vi "MainProgram.vi"() -> ()   [LabVIEW 2015]
uses:
  Semaphores ring.ctl
  Separated VIs/ColorSensors Enum.ctl
  <vilib>/NXT/Subs/ColorSensorColors.ctl
  <vilib>/NXT/Block Support/NXT_InputPort.ctl
  <vilib>/NXT/Block Support/NXT_ButtonSelector.ctl
  Separated VIs/Behavior number ring.ctl
  <vilib>/NXT/Subs/MotorOutput.ctl
  <vilib>/NXT/Block Support/NXT_OutputPort.ctl
  <vilib>/NXT/Dual Mode Library/Advanced/NXTFlag_Assign.vi
  <vilib>/NXT/Dual Mode Library/Advanced/NXTFlag_Get.vi
  <vilib>/NXT/Dual Mode Library/Sensors/Color_Detector.vi
  <vilib>/NXT/Dual Mode Library/Sensors/Sonar_cm.vi
  <vilib>/NXT/Dual Mode Library/Display/drawNumber.vi
  <vilib>/NXT/Dual Mode Library/Sound/Tone.vi
  <vilib>/NXT/NXTIO Xnodes/NXTIONodeSubVIs/NXTMoveMotors.vi
  <vilib>/NXT/NXTIO Xnodes/NXTIONodeSubVIs/NXTStopMotors.vi
  <vilib>/NXT/Dual Mode Library/Waits/Wait_Num.vi
  <vilib>/NXT/Dual Mode Library/Sensors/Touch_Pressed.vi
  <vilib>/NXT/NXTIO Xnodes/NXTIONodeSubVIs/NXTMotorRunDistance.vi
  <vilib>/NXT/NXTIO Xnodes/NXTIONodeSubVIs/NXTMotorSteeringOn.vi
  <vilib>/NXT/Dual Mode Library/Motors/MotorBrake.vi
  <vilib>/NXT/Dual Mode Library/Advanced/NXTFlag_Clear.vi
  <vilib>/NXT/Dual Mode Library/Sensors/readNXTButton.vi
  <vilib>/NXT/NXTIO Xnodes/AddressXNode/NXTIOAddress.xnode
  <vilib>/NXT/NXTIO Xnodes/NXTIOXNode/NXTIO.xnode
  <vilib>/NXT/Subs/LVHSConnector.ctl
  <vilib>/NXT/LegoClasses/BrickReference/BrickReference.lvclass
panel:
  out "Wander Angle":i32
  out "Wander Time":i32
  out "Wander Direction":u16(ring) items=["right", "left"]
  out "Wander Speed":i32
  in  "Behavior Wire In":T1
  in  "Max Behavior Number":i32=8
  in  "Behavior Wires In":T2(array[cluster])
  out "Behavior Wire Output":T1
  out "Behavior Required Found Flag":bool
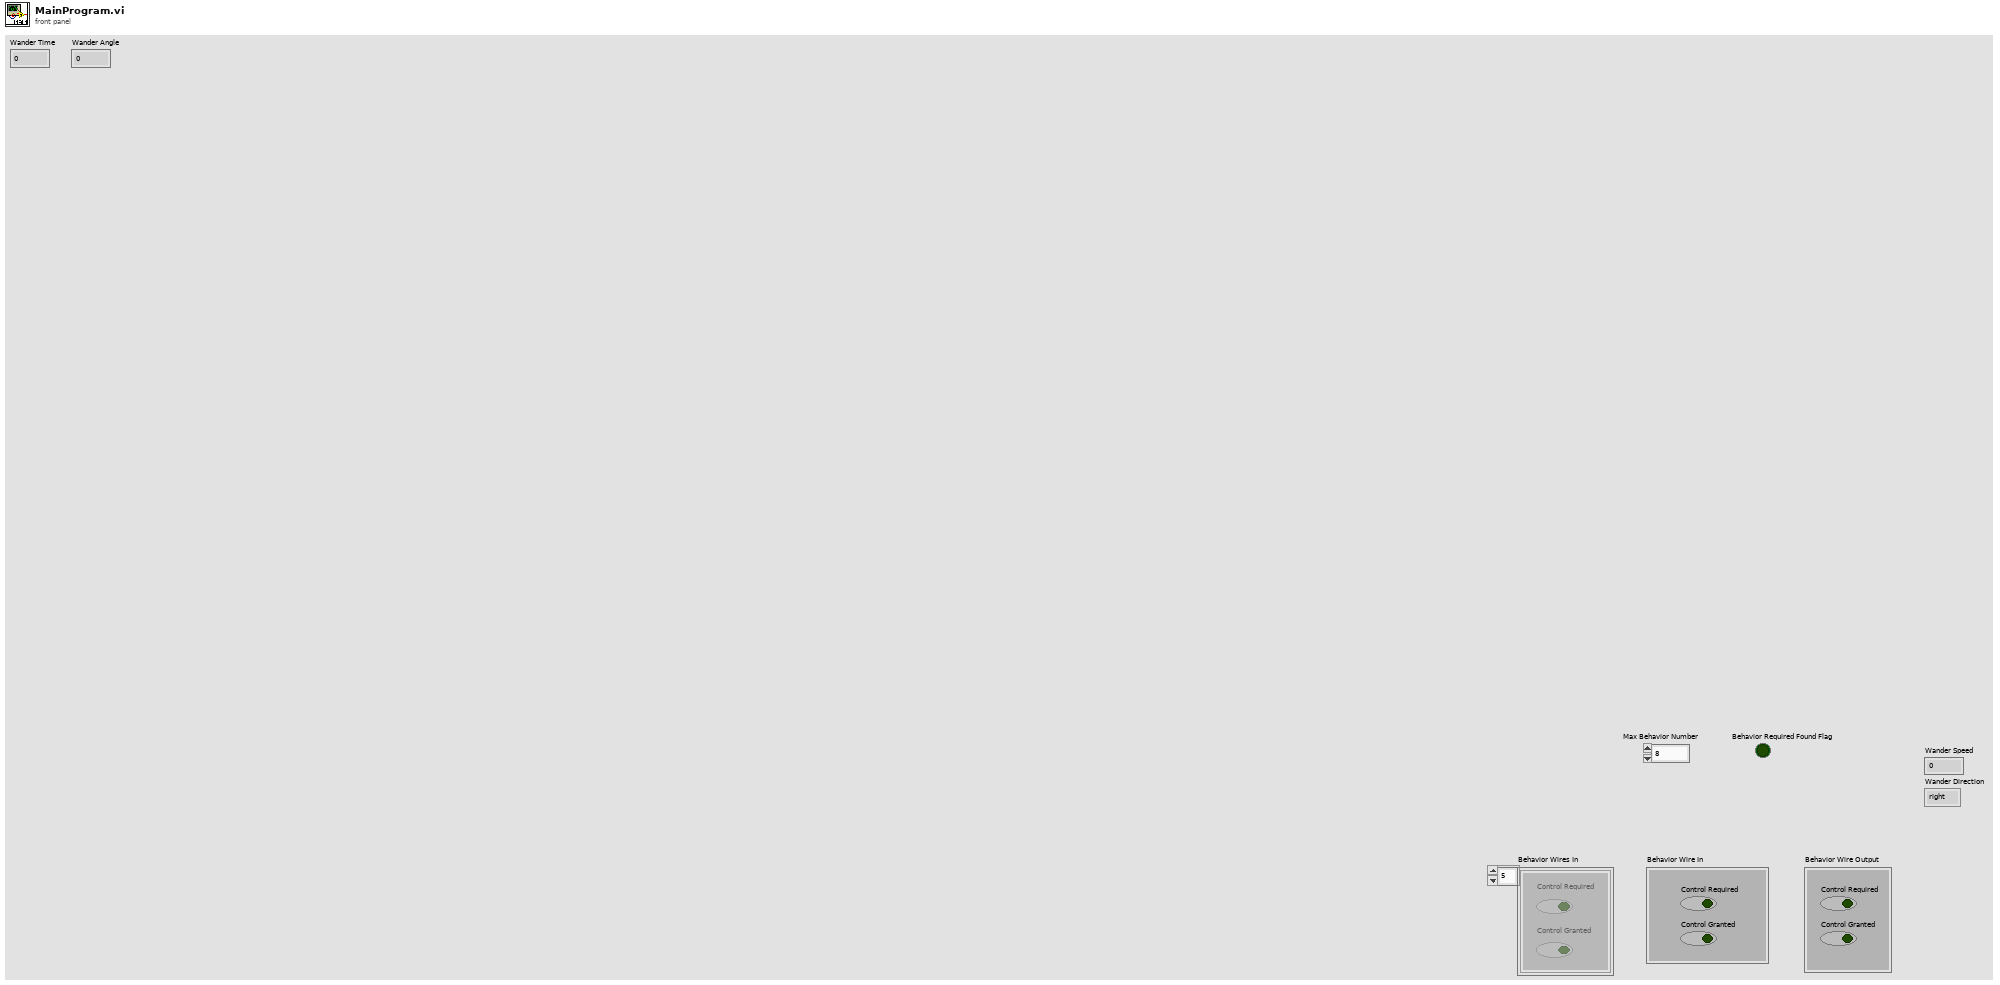
[diagram p1: front panel]
types:
  T1 = cluster{"Control Required":bool, "Control Granted":bool}
  T2 = cluster{"Control Required":bool, "Control Granted":bool}[]
  T3 = typedef "ColorSensors Enum.ctl" = enum16{"Not Recognised", "Black", "Blue", "Green", "Yellow", "Red", "White"}
  T4 = typedef "NXT_OutputPort.ctl" = u8
  T5 = typedef "ColorSensorColors.ctl" = enum16{"No Color", "Black", "Blue", "Green", "Yellow", "Red", "White", "Brown"}
  T6 = typedef "Semaphores ring.ctl" = u16
  T7 = typedef "LVHSConnector.ctl" = refnum<class "BrickReference.lvclass">
  T8 = typedef "NXT_InputPort.ctl" = u32
  T9 = typedef "Behavior number ring.ctl" = u16
  T10 = typedef "MotorOutput.ctl" = u8
  T11 = typedef "NXT_ButtonSelector.ctl" = u16
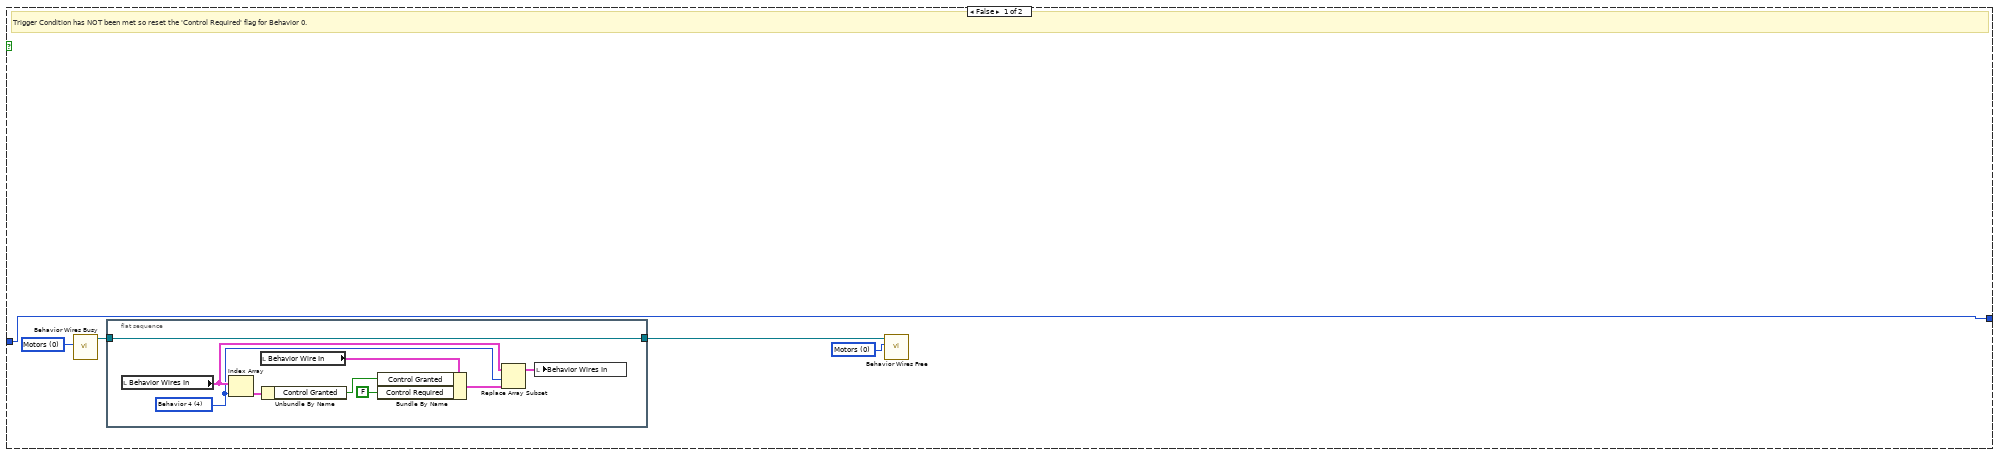
[diagram p3: hidden frame]
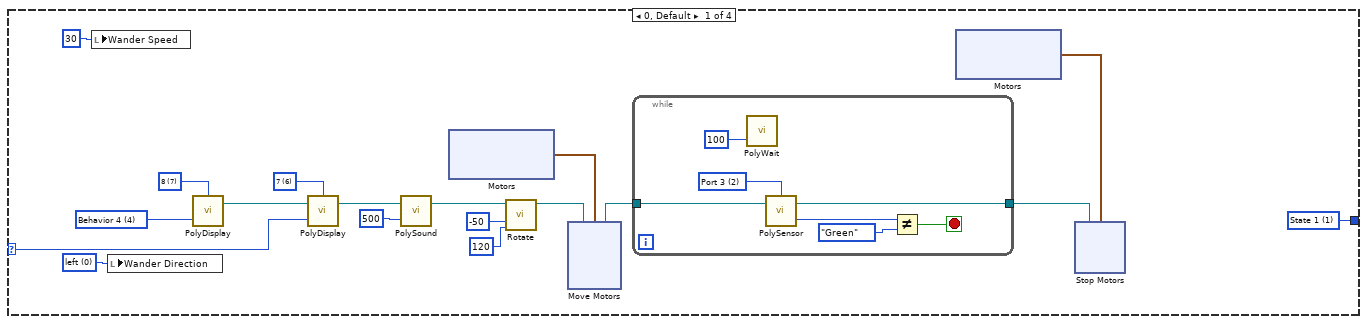
[diagram p5: hidden frame]
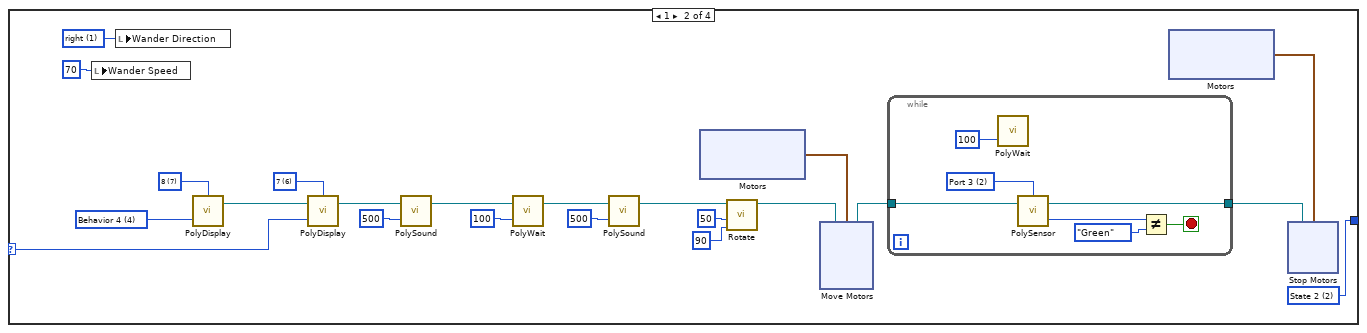
[diagram p6: hidden frame]
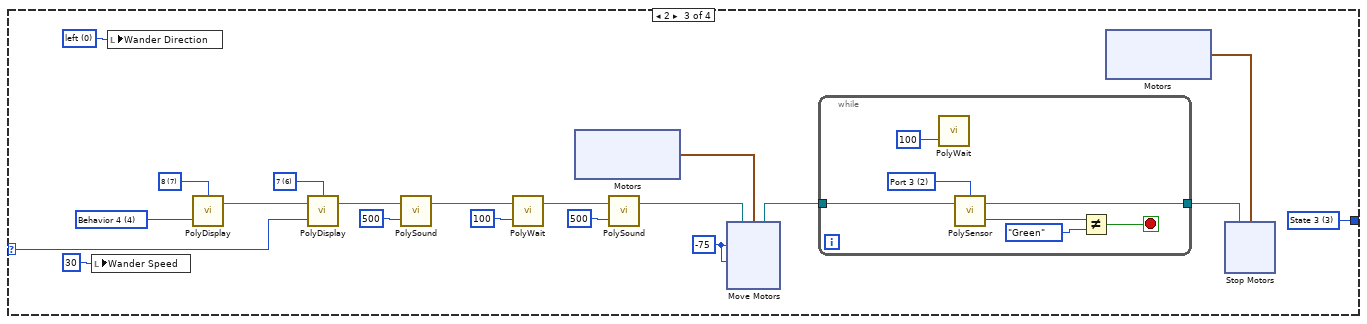
[diagram p7: hidden frame]
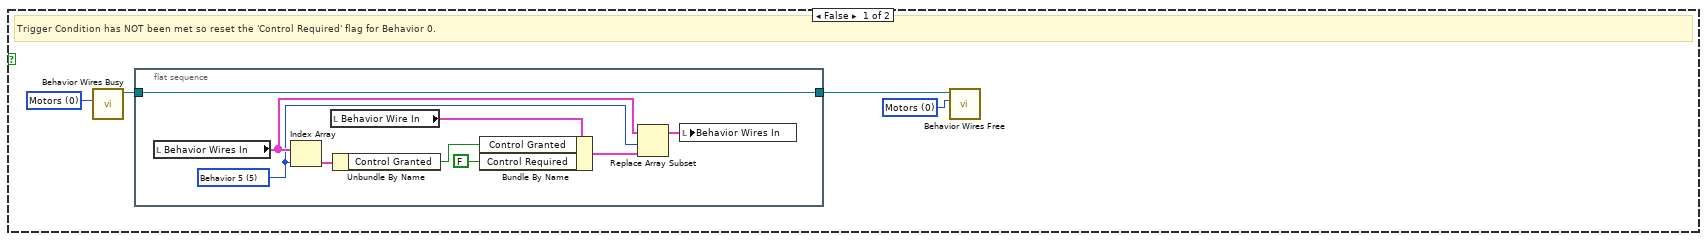
[diagram p8: hidden frame]
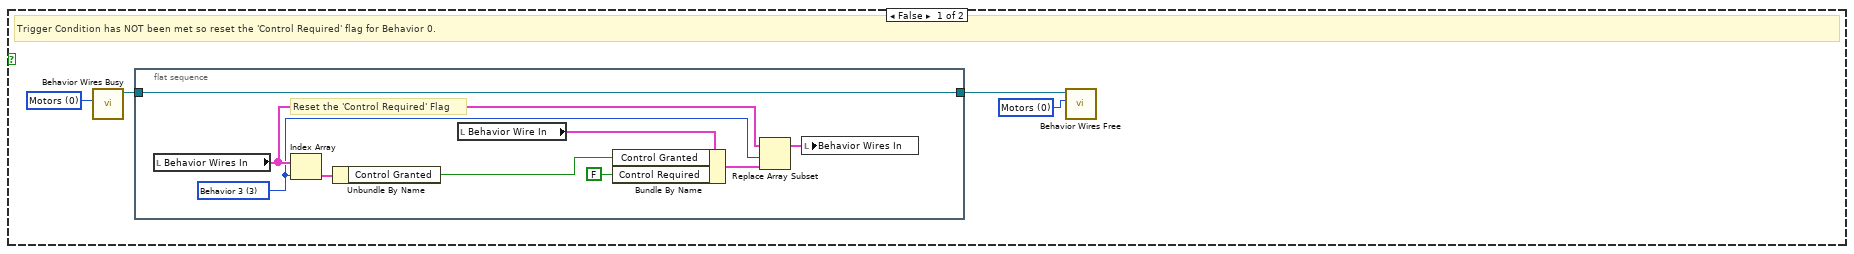
[diagram p10: hidden frame]
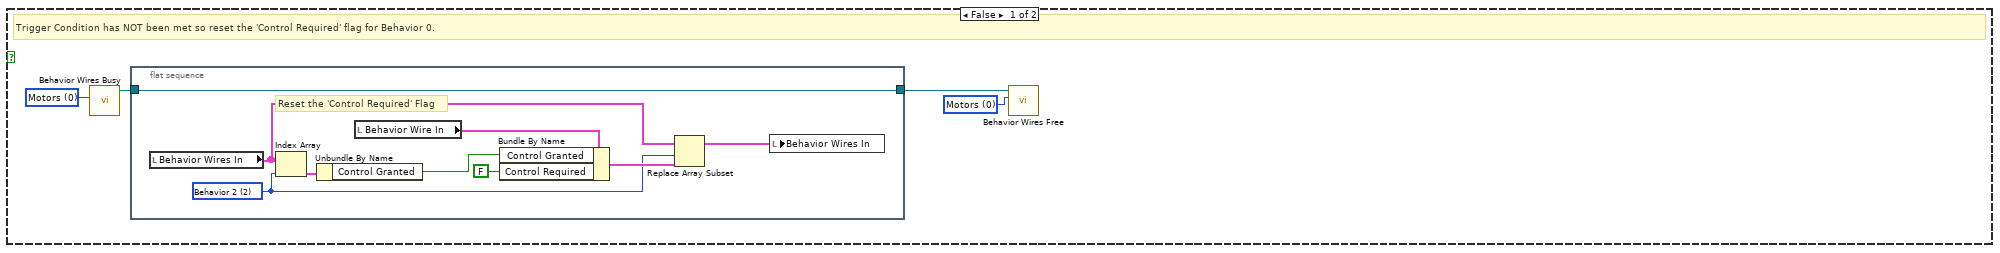
[diagram p12: hidden frame]
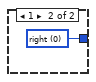
[diagram p14: hidden frame]
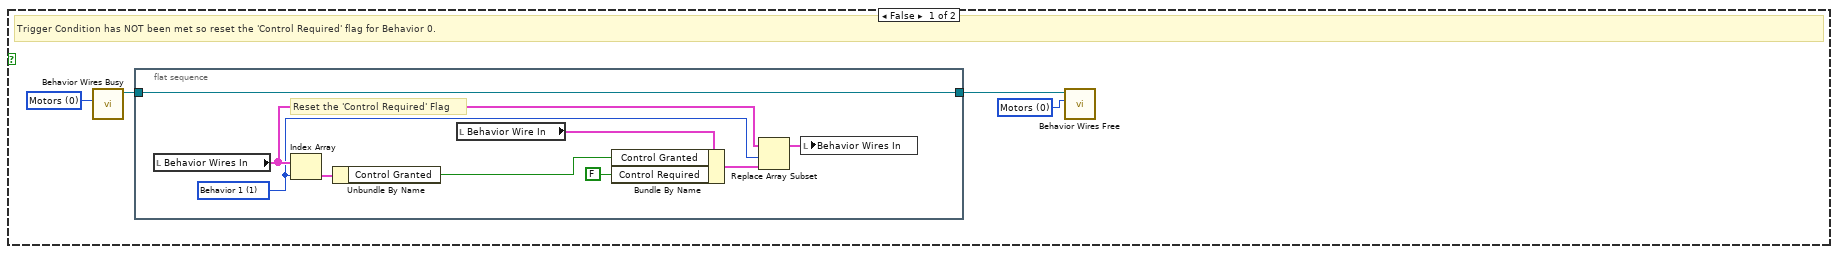
[diagram p15: hidden frame]
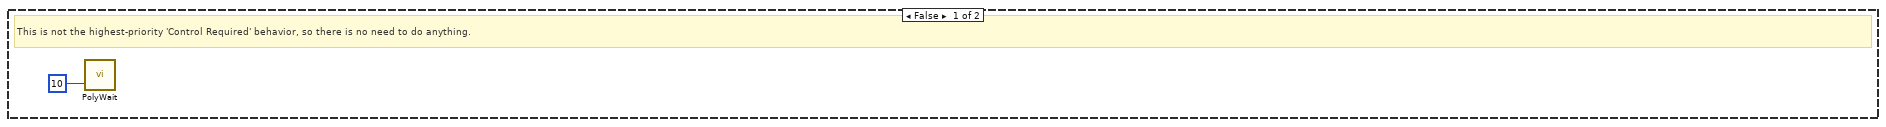
[diagram p17: hidden frame]
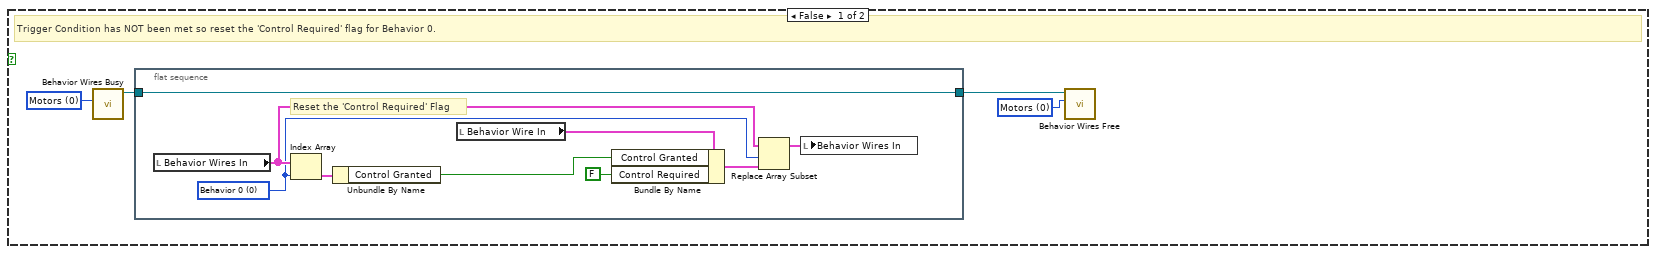
[diagram p20: hidden frame]
diagram:
  n1 = flat-sequence {
    tunnel: [w7] -> w2
    tunnel: w2 -> [w17]
    tunnel: [w18] -> w1
    tunnel: w1 -> [w666]
    frame #0 {
      w5 = u16 1 items=["right", "left"] ("Ring")
      # "Step 1 : Housekeeping\n\nInitalise the Wires array (to False) and \nset the semaphore to begin operation"
      n2 = flat-sequence {
        tunnel: [w13] -> w7
        frame #0 {
          n3 = Initialize Array("Behavior Wire In", "Max Behavior Number") -> (w8:T2)
          n4 = local write "Behavior Wires In"(w8) -> ()
        }
        frame #1 {
          w11 = T6 0 items=["Motors", "Exit", "Sonar"] ("Semaphores")
          w12 = T6 1 items=["Motors", "Exit", "Sonar"] ("Semaphores")
          n5 = call "Behavior Wires Free.vi"("Semaphore Number"=w11) -> ("Sequence Out"=w14:T7)  [unwired: 9 in]
          n6 = call-poly <vilib>:"NXTFlag_Assign_Poly.vi"("Flag State"=FALSE, "NXT/EV3"=w14, "NXT/EV3 Flag Number"=w12) -> ("NXT/EV3"=w13:T7)  [unwired: 1 in]
        }
      }
      "Wander Speed" <- 30
      "Wander Direction" <- w5
      "Wander Time" <- 8
      "Wander Angle" <- 60
    }
    frame #1 {
      w16 = u16 0 items=["State 0", "State 1", "State 2", "State 3"] ("Ring")
      # "Step 2: Execute the behaviors until shutdown is initiated\n                                       \nThe behaviors are placed in separate  parallel loops. \nAccess to the wire cluster array is controlled using a semaphore flag (Contained in 'Behavior Wires Busy' and 'Behavior Wires Free' VIs.. ).\nNote, When 'Behavior Wires Busy' is called, access by the arbiter is suspended,  so it is important that  'Behavior Wires Free' is always called as soon as possible afterwards.\n\nNote: You cannot make a subVI of the Wire operations. The simplified memory manager can't deal with the re-direction.\n\nTo use this example: Behavior 1 - drives in a straight line, Behavior 2 - Sonar at 25 cms rotates and drives off and Behavior 3 - bump sensor causes robot to reverse and pivot"
      n7 = while {
        stop <- w541 stop-if-true
        w540 = T6 1 items=["Motors", "Exit", "Sonar"] ("Semaphores")
        # "Arbiter - Scans all the behaviors to determine which behvior has the highest priority (higher value higher priority). \nCheck from largest index down for 'Control required' Flag set. If first encounter of set flag, set 'Control Granted' flag for behavior.\nReset all lower 'Control Granted' behavior Flags. If no 'Control Required flag' set, reset the resource values"
        n8 = flat-sequence {
          frame #0 {
            # "Reset the 'Behavior Required Found' flag\n before searching..."
            n9 = local write "Behavior Required Found Flag"(FALSE) -> ()
          }
          frame #1 {
            # "... searching for the highest-priority behavior looking for control (i.e. currently with 'Control Required' flag set)."
            n10 = local read "Max Behavior Number"() -> (w543:i32)
            n11 = for {
              N: w543 -> [_]
              i -> [w554]
              n12 = local read "Max Behavior Number"() -> (w545:i32)
              n13 = local read "Behavior Required Found Flag"() -> (w551:bool)
              n14 = local read "Behavior Wires In"() -> (w553:T2)
              n15 = Subtract(x=w545, y=1) -> (x-y=w546:i32)
              n16 = Subtract(x=w546, y=w554) -> (x-y=w549:i32)
              n17 = Index Array(array=w553, index=w549) -> (element=w552:T1)
              n18 = Unbundle By Name(w552) -> ("Control Required"=w548:bool)
              n19 = Not(x=w551) -> (.not. x?=w547:bool)
              n20 = And(x=w547, y=w548) -> (x .and. y?=w550:bool)
              n21 = case shown="True" w550 {
                tunnel: w549 -> [_ w557]
                frame False {
                  # "This is not the highest-priority 'Control Required' behavior, so there is no need to do anything."
                  n22 = call-poly <vilib>:"PolyWait.vi"("Time (100 msec)"=u32 10) -> ()  [unwired: 3 in, 1 out]
                }
                frame True {
                  # "This IS the highest priority 'Control Required' flag"
                  n23 = flat-sequence {
                    tunnel: w557 -> [w563]
                    tunnel: [w563] -> w556
                    tunnel: w556 -> [w569]
                    frame #0 {
                      w558 = T6 0 items=["Motors", "Exit", "Sonar"] ("Semaphores")
                      w559 = T6 0 items=["Motors", "Exit", "Sonar"] ("Semaphores")
                      # "Set the highest 'Control Granted' and 'Behavior Required Found Flag's to True"
                      n24 = flat-sequence {
                        tunnel: w563 -> [w565]
                        tunnel: w561 -> [w564]
                        tunnel: [w564] -> w560
                        frame #0 {
                          n25 = local read "Behavior Wires In"() -> (w567:T2)
                          n26 = Replace Array Subset(array=w567, new element=T1 {"Control Required"=TRUE, "Control Granted"=TRUE} ("Behavior Wire In"), index=w565) -> (w568:T2)
                          n27 = local write "Behavior Wires In"(w568) -> ()
                        }
                      }
                      n28 = local write "Behavior Required Found Flag"(TRUE ("Behavior Required Found Flag")) -> ()
                      n29 = call "Behavior Wires Busy.vi"("Semaphore Number"=w559) -> ("Sequence Out"=w561:T7)  [unwired: 9 in]
                      n30 = call "Behavior Wires Free.vi"("Sequence In"=w560, "Semaphore Number"=w558) -> ()  [unwired: 8 in, 1 out]
                    }
                    frame #1 {
                      # "...And reset all lower 'Control Granted' Flags"
                      n31 = for {
                        N: w569 -> [_]
                        tunnel: w569 -> [w572]
                        i -> [w570]
                        n32 = Not Equal?(x=w572, y=w570) -> (x != y?=w571:bool)
                        n33 = case shown="True" w571 {
                          tunnel: w570 -> [_ w575]
                          frame False {
                            # "This is the highest priority index so DO NOT reset the 'Control Granted' flag."
                          }
                          frame True {
                            w573 = T6 0 items=["Motors", "Exit", "Sonar"] ("Semaphores")
                            w574 = T6 0 items=["Motors", "Exit", "Sonar"] ("Semaphores")
                            # "This is NOT the highest priority index so DO reset the 'Control Granted' flag."
                            n34 = call "Behavior Wires Busy.vi"("Semaphore Number"=w574) -> ("Sequence Out"=w576:T7)  [unwired: 9 in]
                            n35 = flat-sequence {
                              tunnel: w575 -> [w579]
                              tunnel: [w578] -> w577
                              tunnel: w576 -> [w578]
                              frame #0 {
                                # "Reset 'Control Granted' flag for remaining behaviors"
                                n36 = local read "Behavior Wires In"() -> (w584:T2)
                                n37 = Index Array(array=w584, index=w579) -> (element=w582:T1)
                                n38 = Unbundle By Name(w582) -> ("Control Required"=w581:bool)
                                n39 = local read "Behavior Wire In"() -> (w583:T1)
                                n40 = Bundle By Name(cluster=w583, "Control Required"=w581, "Control Granted"=FALSE) -> (w585:T1)
                                n41 = Replace Array Subset(array=w584, new element=w585, index=w579) -> (w586:T2)
                                n42 = local write "Behavior Wires In"(w586) -> ()
                              }
                            }
                            n43 = call "Behavior Wires Free.vi"("Sequence In"=w577, "Semaphore Number"=w573) -> ()  [unwired: 8 in, 1 out]
                          }
                        }
                      }
                    }
                  }
                }
              }
            }
          }
        }
        n44 = call-poly <vilib>:"NXTFlag_Get_Poly.vi"("NXT/EV3 Flag Number"=w540) -> ("status"=w541:bool)  [unwired: 2 in, 1 out]
      }
      n45 = while {
        stop <- w482 stop-if-true
        w473 = T8 3 items=["Port 1", "Port 2", "Port 3", "Port 4"] ("Port (Port 4)")
        w474 = T8 2 items=["Port 1", "Port 2", "Port 3", "Port 4"] ("Port (Port 3)")
        w481 = T6 1 items=["Motors", "Exit", "Sonar"] ("Semaphores")
        # "No color -> Change to some color"
        # "Behavior 1"
        n46 = call-poly <vilib>:"PolySensor.vi"("Port (Port 3)"=w474) -> ("Detected Color"=w480:T5)  [unwired: 2 in, 1 out]
        n47 = call-poly <vilib>:"PolySensor.vi"("Port (Port 4)"=w473) -> ("Distance (cm)"=w477:i16)  [unwired: 2 in, 1 out]
        n48 = Equal?(x=w480, y=ColorSensorColors."White") -> (x = y?=w478:bool)
        n49 = Less?(x=w477, y=i16 10) -> (x < y?=w475:bool)
        n50 = And(x=w475, y=w478) -> (x .and. y?=w472:bool)
        n51 = case shown="True" w472 {
          frame False {
            w483 = T6 0 items=["Motors", "Exit", "Sonar"] ("Semaphores")
            w484 = T6 0 items=["Motors", "Exit", "Sonar"] ("Semaphores")
            # "Trigger Condition has NOT been met so reset the 'Control Required' flag for Behavior 0."
            n52 = call "Behavior Wires Busy.vi"("Semaphore Number"=w483) -> ("Sequence Out"=w485:T7)  [unwired: 9 in]
            n53 = flat-sequence {
              tunnel: w485 -> [w487]
              tunnel: [w487] -> w486
              frame #0 {
                w490 = T9 1 items=["Behavior 0", "Behavior 1", "Behavior 2", "Behavior 3", "Behavior 4", "Behavior 5", "Behavior 6"] ("Ring")
                # "Reset the 'Control Required' Flag"
                n54 = local read "Behavior Wires In"() -> (w492:T2)
                n55 = Index Array(array=w492, index=w490) -> (element=w495:T1)
                n56 = Unbundle By Name(w495) -> ("Control Granted"=w488:bool)
                n57 = local read "Behavior Wire In"() -> (w494:T1)
                n58 = Bundle By Name(cluster=w494, "Control Granted"=w488, "Control Required"=FALSE) -> (w491:T1)
                n59 = Replace Array Subset(array=w492, new element=w491, index=w490) -> (w489:T2)
                n60 = local write "Behavior Wires In"(w489) -> ()
              }
            }
            n61 = call "Behavior Wires Free.vi"("Sequence In"=w486, "Semaphore Number"=w484) -> ()  [unwired: 8 in, 1 out]
          }
          frame True {
            w496 = T6 0 items=["Motors", "Exit", "Sonar"] ("Semaphores")
            w497 = T6 0 items=["Motors", "Exit", "Sonar"] ("Semaphores")
            # "Trigger condition has been  met so set 'Control Required' Flag and execute behavior if 'Control Granted' flag for Behavior 1 is set."
            n62 = call "Behavior Wires Busy.vi"("Semaphore Number"=w497) -> ("Sequence Out"=w500:T7)  [unwired: 9 in]
            n63 = flat-sequence {
              tunnel: w500 -> [w502]
              tunnel: [w502] -> w499
              tunnel: [w501] -> w498
              frame #0 {
                w508 = T9 1 items=["Behavior 0", "Behavior 1", "Behavior 2", "Behavior 3", "Behavior 4", "Behavior 5", "Behavior 6"] ("Ring")
                # "Trigger Condition Met"
                # "Step 2: Since trigger Condition has been met, set the 'Control Required' flag for this behavior"
                n64 = local read "Behavior Wires In"() -> (w506:T2)
                n65 = Index Array(array=w506, index=w508) -> (element=w504:T1)
                n66 = local read "Behavior Wire In"() -> (w505:T1)
                n67 = Unbundle By Name(w504) -> ("Control Granted"=w501:bool)
                n68 = Bundle By Name(cluster=w505, "Control Required"=TRUE ("Control Granted"), "Control Granted"=w501) -> (w507:T1)
                n69 = Replace Array Subset(array=w506, new element=w507, index=w508) -> (w509:T2)
                n70 = local write "Behavior Wires In"(w509) -> ()
              }
            }
            n71 = call "Behavior Wires Free.vi"("Sequence In"=w499, "Semaphore Number"=w496) -> ()  [unwired: 8 in, 1 out]
            n72 = case shown="True" w498 {
              frame False {
                # "Control has NOT been granted to this Behavior, so do nothing."
              }
              frame True {
                w515 = T9 1 items=["Behavior 0", "Behavior 1", "Behavior 2", "Behavior 3", "Behavior 4", "Behavior 5", "Behavior 6"] ("Ring")
                w521 = u16 0 items=["right", "left"] ("Ring")
                w533 = i16 7 items=["1", "2", "3", "4", "5", "6", "7", "8", "9", "10", "11", "12"] ("Line")
                # "Your code for Behavior 1 replaces the code here"
                n73 = xnode "Motors"() -> ("Motor"=w522:cluster{"Port":T4, "Port":T4})
                n74 = call-poly <vilib>:"PolyDisplay.vi"("number"=w515, "Line"=w533) -> ("NXT/EV3"=w524:T7)  [unwired: 2 in]
                n75 = xnode "Stop Motors"("Motors"=w522, "NXT/EV3"=w524) -> ("NXT/EV3"=w523:T7)
                n76 = call-poly <vilib>:"PolySound.vi"("Duration (500 ms)"=u16 500, "NXT/EV3"=w523) -> ("NXT/EV3"=w532:T7)  [unwired: 2 in]
                n77 = call <vilib>:"RandomNumber.vi"("Max Value"=u16 2) -> ("Random Number"=w519:u16)  [unwired: 2 in, 1 out]
                n78 = call-poly <vilib>:"PolyWait.vi"("Time (100 msec)"=u32 500, "NXT/EV3"=w532) -> ("NXT/EV3"=w529:T7)  [unwired: 2 in]
                n79 = Equal?(x=w519, y=w521) -> (x = y?=w520:bool)
                n80 = call <vilib>:"RandomNumber.vi"("Max Value"=u16 60) -> ("Random Number"=w511:u16)  [unwired: 2 in, 1 out]
                n81 = Select(t=u16 1, s=w520, f=i16 -1) -> (s? t:f=w517:u16)
                n82 = call-poly <vilib>:"PolySound.vi"("Duration (500 ms)"=u16 500, "NXT/EV3"=w529) -> ("NXT/EV3"=w514:T7)  [unwired: 2 in]
                n83 = Multiply(x=i16 70 ("Direction/Speed"), y=w517) -> (x*y=w513:u16)
                n84 = Add(x=w511, y=120) -> (x+y=w512:i32)
                n85 = call "Rotate.vi"("Rotation"=w512, "Direction/Speed"=w513, "Input"=w514) -> ()  [unwired: 8 in, 1 out]
              }
            }
          }
        }
        n86 = call-poly <vilib>:"NXTFlag_Get_Poly.vi"("NXT/EV3 Flag Number"=w481) -> ("status"=w482:bool)  [unwired: 2 in, 1 out]
      }
      n87 = while {
        shift-right: [w45] -> _
        shift-left: w16 -> [w46]
        stop <- w48 stop-if-true
        w38 = T8 3 items=["Port 1", "Port 2", "Port 3", "Port 4"] ("Port (Port 4)")
        w35 = T8 2 items=["Port 1", "Port 2", "Port 3", "Port 4"] ("Port (Port 3)")
        w47 = T6 1 items=["Motors", "Exit", "Sonar"] ("Semaphores")
        # "Behavior 4"
        n88 = call-poly <vilib>:"PolySensor.vi"("Port (Port 3)"=w35) -> ("Detected Color"=w34:T5)  [unwired: 2 in, 1 out]
        n89 = call-poly <vilib>:"PolySensor.vi"("Port (Port 4)"=w38) -> ("Distance (cm)"=w39:i16)  [unwired: 2 in, 1 out]
        n90 = Greater Or Equal?(x=w39, y=i16 7) -> (x >= y?=w42:bool)
        n91 = Less Or Equal?(x=w39, y=i16 12) -> (x <= y?=w43:bool)
        n92 = Equal?(x=w34, y=ColorSensors_Enum."Green" ("ColorSensor Colours")) -> (x = y?=w37:bool)
        n93 = And(x=w42, y=w43) -> (x .and. y?=w44:bool)
        n94 = And(x=w37, y=w44) -> (x .and. y?=w33:bool)
        n95 = case shown="True" w33 {
          tunnel: w46 -> [w49 w64]
          tunnel: [w49 w63] -> w45
          frame False {
            w50 = T6 0 items=["Motors", "Exit", "Sonar"] ("Semaphores")
            w51 = T6 0 items=["Motors", "Exit", "Sonar"] ("Semaphores")
            # "Trigger Condition has NOT been met so reset the 'Control Required' flag for Behavior 0."
            n96 = call "Behavior Wires Busy.vi"("Semaphore Number"=w50) -> ("Sequence Out"=w52:T7)  [unwired: 9 in]
            n97 = flat-sequence {
              tunnel: w52 -> [w54]
              tunnel: [w54] -> w53
              frame #0 {
                w57 = T9 4 items=["Behavior 0", "Behavior 1", "Behavior 2", "Behavior 3", "Behavior 4", "Behavior 5", "Behavior 6"] ("Ring")
                n98 = local read "Behavior Wires In"() -> (w59:T2)
                n99 = Index Array(array=w59, index=w57) -> (element=w62:T1)
                n100 = local read "Behavior Wire In"() -> (w61:T1)
                n101 = Unbundle By Name(w62) -> ("Control Granted"=w55:bool)
                n102 = Bundle By Name(cluster=w61, "Control Granted"=w55, "Control Required"=FALSE) -> (w58:T1)
                n103 = Replace Array Subset(array=w59, new element=w58, index=w57) -> (w56:T2)
                n104 = local write "Behavior Wires In"(w56) -> ()
              }
            }
            n105 = call "Behavior Wires Free.vi"("Sequence In"=w53, "Semaphore Number"=w51) -> ()  [unwired: 8 in, 1 out]
          }
          frame True {
            w65 = T6 0 items=["Motors", "Exit", "Sonar"] ("Semaphores")
            w66 = T6 0 items=["Motors", "Exit", "Sonar"] ("Semaphores")
            # "Trigger condition has been  met so set 'Control Required' Flag and execute behavior if 'Control Granted' flag for Behavior 4 is set."
            n106 = call "Behavior Wires Busy.vi"("Semaphore Number"=w66) -> ("Sequence Out"=w69:T7)  [unwired: 9 in]
            n107 = flat-sequence {
              tunnel: w69 -> [w71]
              tunnel: [w71] -> w68
              tunnel: [w70] -> w67
              frame #0 {
                w77 = T9 4 items=["Behavior 0", "Behavior 1", "Behavior 2", "Behavior 3", "Behavior 4", "Behavior 5", "Behavior 6"] ("Ring")
                # "Step 2: Since trigger Condition has been met, set the 'Control Required' flag for this behavior"
                n108 = local read "Behavior Wires In"() -> (w75:T2)
                n109 = Index Array(array=w75, index=w77) -> (element=w73:T1)
                n110 = local read "Behavior Wire In"() -> (w74:T1)
                n111 = Unbundle By Name(w73) -> ("Control Granted"=w70:bool)
                n112 = Bundle By Name(cluster=w74, "Control Required"=TRUE ("Control Granted"), "Control Granted"=w70) -> (w76:T1)
                n113 = Replace Array Subset(array=w75, new element=w76, index=w77) -> (w78:T2)
                n114 = local write "Behavior Wires In"(w78) -> ()
              }
            }
            n115 = call "Behavior Wires Free.vi"("Sequence In"=w68, "Semaphore Number"=w65) -> ()  [unwired: 8 in, 1 out]
            n116 = case shown="True" w67 {
              tunnel: w64 -> [w79 w81]
              tunnel: [w79 w80] -> w63
              frame False {
                # "Control has NOT been granted to this Behavior, so do nothing."
              }
              frame True {
                # "Your code for Behavior 4 replaces the code here"
                n117 = case shown="3" w81 {
                  selector: w81 -> [w87 w132 w173 w208]
                  tunnel: [w86 w131 w174 w218] -> w80
                  frame 0, Default {
                    w83 = u16 0 items=["left", "right"] ("Ring")
                    w85 = T9 4 items=["Behavior 0", "Behavior 1", "Behavior 2", "Behavior 3", "Behavior 4", "Behavior 5", "Behavior 6"] ("Ring")
                    w86 = u16 1 items=["State 0", "State 1", "State 2", "State 3"] ("Ring")
                    w98 = i16 7 items=["1", "2", "3", "4", "5", "6", "7", "8", "9", "10", "11", "12"] ("Line")
                    w99 = i16 6 items=["1", "2", "3", "4", "5", "6", "7", "8", "9", "10", "11", "12"] ("Line")
                    n118 = local write "Wander Speed"(i16 30 ("Wander Speed")) -> ()
                    n119 = local write "Wander Direction"(w83) -> ()
                    n120 = call-poly <vilib>:"PolyDisplay.vi"("number"=w85, "Line"=w98) -> ("NXT/EV3"=w97:T7)  [unwired: 2 in]
                    n121 = call-poly <vilib>:"PolyDisplay.vi"("number"=w87, "NXT/EV3"=w97, "Line"=w99) -> ("NXT/EV3"=w96:T7)  [unwired: 1 in]
                    n122 = call-poly <vilib>:"PolySound.vi"("Duration (500 ms)"=u16 500, "NXT/EV3"=w96) -> ("NXT/EV3"=w94:T7)  [unwired: 2 in]
                    n123 = xnode "Motors"() -> ("Motor"=w91:cluster{"Port":T4, "Port":T4})
                    n124 = call "Rotate.vi"("Rotation"=i16 120, "Direction/Speed"=i16 -50, "Input"=w94) -> ("Output"=w92:T7)  [unwired: 8 in]
                    n125 = xnode "Move Motors"("Motors"=w91, "NXT/EV3"=w92) -> ("NXT/EV3"=w90:T7)  [unwired: 2 in]
                    n126 = while {
                      tunnel: w90 -> [w112]
                      tunnel: [w107] -> w89
                      stop <- w108 stop-if-true
                      w111 = T8 2 items=["Port 1", "Port 2", "Port 3", "Port 4"] ("Port (Port 3)")
                      n127 = call-poly <vilib>:"PolyWait.vi"("Time (100 msec)"=u32 100) -> ()  [unwired: 3 in, 1 out]
                      n128 = call-poly <vilib>:"PolySensor.vi"("NXT/EV3"=w112, "Port (Port 3)"=w111) -> ("Detected Color"=w110:T5, "NXT/EV3"=w107:T7)  [unwired: 1 in]
                      n129 = Not Equal?(x=w110, y=ColorSensorColors."Green" ("Detected Color")) -> (x != y?=w108:bool)
                    }
                    n130 = xnode "Motors"() -> ("Motor"=w88:cluster{"Port":T4, "Port":T4})
                    n131 = xnode "Stop Motors"("Motors"=w88, "NXT/EV3"=w89) -> ()  [unwired: 1 out]
                  }
                  frame 1 {
                    w126 = u16 1 items=["left", "right"] ("Wander Direction")
                    w128 = T9 4 items=["Behavior 0", "Behavior 1", "Behavior 2", "Behavior 3", "Behavior 4", "Behavior 5", "Behavior 6"] ("Ring")
                    w131 = u16 2 items=["State 0", "State 1", "State 2", "State 3"] ("Ring")
                    w134 = i16 7 items=["1", "2", "3", "4", "5", "6", "7", "8", "9", "10", "11", "12"] ("Line")
                    w133 = i16 6 items=["1", "2", "3", "4", "5", "6", "7", "8", "9", "10", "11", "12"] ("Line")
                    n132 = local write "Wander Speed"(i16 70 ("Wander Speed")) -> ()
                    n133 = local write "Wander Direction"(w126) -> ()
                    n134 = call-poly <vilib>:"PolyDisplay.vi"("number"=w128, "Line"=w134) -> ("NXT/EV3"=w135:T7)  [unwired: 2 in]
                    n135 = call-poly <vilib>:"PolyDisplay.vi"("number"=w132, "NXT/EV3"=w135, "Line"=w133) -> ("NXT/EV3"=w136:T7)  [unwired: 1 in]
                    n136 = call-poly <vilib>:"PolySound.vi"("Duration (500 ms)"=u16 500, "NXT/EV3"=w136) -> ("NXT/EV3"=w123:T7)  [unwired: 2 in]
                    n137 = call-poly <vilib>:"PolyWait.vi"("Time (100 msec)"=u32 100, "NXT/EV3"=w123) -> ("NXT/EV3"=w122:T7)  [unwired: 2 in]
                    n138 = call-poly <vilib>:"PolySound.vi"("Duration (500 ms)"=u16 500, "NXT/EV3"=w122) -> ("NXT/EV3"=w129:T7)  [unwired: 2 in]
                    n139 = xnode "Motors"() -> ("Motor"=w140:cluster{"Port":T4, "Port":T4})
                    n140 = call "Rotate.vi"("Rotation"=i16 90, "Direction/Speed"=i16 50, "Input"=w129) -> ("Output"=w139:T7)  [unwired: 8 in]
                    n141 = xnode "Move Motors"("Motors"=w140, "NXT/EV3"=w139) -> ("NXT/EV3"=w141:T7)  [unwired: 2 in]
                    n142 = while {
                      tunnel: w141 -> [w156]
                      tunnel: [w151] -> w142
                      stop <- w152 stop-if-true
                      w155 = T8 2 items=["Port 1", "Port 2", "Port 3", "Port 4"] ("Port (Port 3)")
                      n143 = call-poly <vilib>:"PolyWait.vi"("Time (100 msec)"=u32 100) -> ()  [unwired: 3 in, 1 out]
                      n144 = call-poly <vilib>:"PolySensor.vi"("NXT/EV3"=w156, "Port (Port 3)"=w155) -> ("Detected Color"=w154:T5, "NXT/EV3"=w151:T7)  [unwired: 1 in]
                      n145 = Not Equal?(x=w154, y=ColorSensorColors."Green" ("Detected Color")) -> (x != y?=w152:bool)
                    }
                    n146 = xnode "Motors"() -> ("Motor"=w143:cluster{"Port":T4, "Port":T4})
                    n147 = xnode "Stop Motors"("Motors"=w143, "NXT/EV3"=w142) -> ()  [unwired: 1 out]
                  }
                  frame 2 {
                    w169 = i8 -75 ("Power/Speed 1")
                    w171 = u16 0 items=["left", "right"] ("Wander Direction")
                    w172 = T9 4 items=["Behavior 0", "Behavior 1", "Behavior 2", "Behavior 3", "Behavior 4", "Behavior 5", "Behavior 6"] ("Ring")
                    w174 = u16 3 items=["State 0", "State 1", "State 2", "State 3"] ("Ring")
                    w178 = i16 7 items=["1", "2", "3", "4", "5", "6", "7", "8", "9", "10", "11", "12"] ("Line")
                    w177 = i16 6 items=["1", "2", "3", "4", "5", "6", "7", "8", "9", "10", "11", "12"] ("Line")
                    n148 = local write "Wander Speed"(i16 30 ("Wander Speed")) -> ()
                    n149 = local write "Wander Direction"(w171) -> ()
                    n150 = call-poly <vilib>:"PolyDisplay.vi"("number"=w172, "Line"=w178) -> ("NXT/EV3"=w179:T7)  [unwired: 2 in]
                    n151 = call-poly <vilib>:"PolyDisplay.vi"("number"=w173, "NXT/EV3"=w179, "Line"=w177) -> ("NXT/EV3"=w180:T7)  [unwired: 1 in]
                    n152 = call-poly <vilib>:"PolySound.vi"("Duration (500 ms)"=u16 500, "NXT/EV3"=w180) -> ("NXT/EV3"=w168:T7)  [unwired: 2 in]
                    n153 = call-poly <vilib>:"PolyWait.vi"("Time (100 msec)"=u32 100, "NXT/EV3"=w168) -> ("NXT/EV3"=w167:T7)  [unwired: 2 in]
                    n154 = xnode "Motors"() -> ("Motor"=w182:cluster{"Port":T4, "Port":T4})
                    n155 = call-poly <vilib>:"PolySound.vi"("Duration (500 ms)"=u16 500, "NXT/EV3"=w167) -> ("NXT/EV3"=w175:T7)  [unwired: 2 in]
                    n156 = xnode "Move Motors"("Power/Speed 2"=w169, "Power/Speed 1"=w169, "Motors"=w182, "NXT/EV3"=w175) -> ("NXT/EV3"=w183:T7)
                    n157 = while {
                      tunnel: w183 -> [w198]
                      tunnel: [w193] -> w184
                      stop <- w194 stop-if-true
                      w197 = T8 2 items=["Port 1", "Port 2", "Port 3", "Port 4"] ("Port (Port 3)")
                      n158 = call-poly <vilib>:"PolyWait.vi"("Time (100 msec)"=u32 100) -> ()  [unwired: 3 in, 1 out]
                      n159 = call-poly <vilib>:"PolySensor.vi"("NXT/EV3"=w198, "Port (Port 3)"=w197) -> ("Detected Color"=w196:T5, "NXT/EV3"=w193:T7)  [unwired: 1 in]
                      n160 = Not Equal?(x=w196, y=ColorSensorColors."Green" ("Detected Color")) -> (x != y?=w194:bool)
                    }
                    n161 = xnode "Motors"() -> ("Motor"=w185:cluster{"Port":T4, "Port":T4})
                    n162 = xnode "Stop Motors"("Motors"=w185, "NXT/EV3"=w184) -> ()  [unwired: 1 out]
                  }
                  frame 3 {
                    w209 = u16 1 items=["left", "right"] ("Ring")
                    w210 = u16 0 items=["left", "right"] ("Ring")
                    w211 = u16 1 items=["left", "right"] ("Ring")
                    w217 = T9 4 items=["Behavior 0", "Behavior 1", "Behavior 2", "Behavior 3", "Behavior 4", "Behavior 5", "Behavior 6"] ("Ring")
                    w219 = u16 1 items=["State 0", "State 1", "State 2", "State 3"] ("Ring")
                    w223 = T8 3 items=["Port 1", "Port 2", "Port 3", "Port 4"] ("Port (Port 4)")
                    w220 = u16 2 items=["State 0", "State 1", "State 2", "State 3"] ("Ring")
                    w233 = i16 7 items=["1", "2", "3", "4", "5", "6", "7", "8", "9", "10", "11", "12"] ("Line")
                    w232 = i16 6 items=["1", "2", "3", "4", "5", "6", "7", "8", "9", "10", "11", "12"] ("Line")
                    n163 = call <vilib>:"RandomNumber.vi"("Max Value"=u16 2) -> ("Random Number"=w214:u16)  [unwired: 2 in, 1 out]
                    n164 = local write "Wander Speed"(i16 50 ("Wander Speed")) -> ()
                    n165 = Equal?(x=w214, y=w209) -> (x = y?=w213:bool)
                    n166 = call-poly <vilib>:"PolyDisplay.vi"("number"=w217, "Line"=w233) -> ("NXT/EV3"=w234:T7)  [unwired: 2 in]
                    n167 = xnode "Motors"() -> ("Motor"=w235:cluster{"Port":T4, "Port":T4})
                    n168 = Select(t=w211, s=w213, f=w210) -> (s? t:f=w212:u16)
                    n169 = call-poly <vilib>:"PolyDisplay.vi"("number"=w208, "NXT/EV3"=w234, "Line"=w232) -> ("NXT/EV3"=w231:T7)  [unwired: 1 in]
                    n170 = local write "Wander Direction"(w212) -> ()
                    n171 = xnode "Move Motors"("Power/Speed 2"=i8 -50, "Power/Speed 1"=i8 -75, "Motors"=w235, "NXT/EV3"=w231) -> ("NXT/EV3"=w228:T7)
                    n172 = xnode "Motors"() -> ("Motor"=w236:cluster{"Port":T4, "Port":T4})
                    n173 = call-poly <vilib>:"PolyWait.vi"("Time (1 sec)"=i16 3, "NXT/EV3"=w228) -> ("NXT/EV3"=w226:T7)  [unwired: 2 in]
                    n174 = xnode "Stop Motors"("Motors"=w236, "NXT/EV3"=w226) -> ("NXT/EV3"=w225:T7)
                    n175 = call-poly <vilib>:"PolySensor.vi"("NXT/EV3"=w225, "Port (Port 4)"=w223) -> ("Distance (cm)"=w224:i16)  [unwired: 1 in, 1 out]
                    n176 = Less Or Equal?(x=w224, y=i16 10) -> (x <= y?=w221:bool)
                    n177 = Select(t=w220, s=w221, f=w219) -> (s? t:f=w218:u16)
                  }
                }
              }
            }
          }
        }
        n178 = call-poly <vilib>:"NXTFlag_Get_Poly.vi"("NXT/EV3 Flag Number"=w47) -> ("status"=w48:bool)  [unwired: 2 in, 1 out]
      }
      n179 = while {
        stop <- w265 stop-if-true
        w258 = T8 3 items=["Port 1", "Port 2", "Port 3", "Port 4"] ("Port (Port 4)")
        w256 = T8 2 items=["Port 1", "Port 2", "Port 3", "Port 4"] ("Port (Port 3)")
        w264 = T6 1 items=["Motors", "Exit", "Sonar"] ("Semaphores")
        # "Behavior 5"
        n180 = call-poly <vilib>:"PolySensor.vi"("Port (Port 4)"=w258) -> ("Distance (cm)"=w259:i16)  [unwired: 2 in, 1 out]
        n181 = call-poly <vilib>:"PolySensor.vi"("Port (Port 3)"=w256) -> ("Detected Color"=w255:T5)  [unwired: 2 in, 1 out]
        n182 = Greater Or Equal?(x=w259, y=i16 7) -> (x >= y?=w262:bool)
        n183 = Less Or Equal?(x=w259, y=i16 12) -> (x <= y?=w263:bool)
        n184 = Equal?(x=w255, y=ColorSensors_Enum."Red" ("ColorSensor Colours")) -> (x = y?=w254:bool)
        n185 = And(x=w262, y=w263) -> (x .and. y?=w253:bool)
        n186 = And(x=w253, y=w254) -> (x .and. y?=w252:bool)
        n187 = case shown="True" w252 {
          frame False {
            w266 = T6 0 items=["Motors", "Exit", "Sonar"] ("Semaphores")
            w267 = T6 0 items=["Motors", "Exit", "Sonar"] ("Semaphores")
            # "Trigger Condition has NOT been met so reset the 'Control Required' flag for Behavior 0."
            n188 = call "Behavior Wires Busy.vi"("Semaphore Number"=w266) -> ("Sequence Out"=w268:T7)  [unwired: 9 in]
            n189 = flat-sequence {
              tunnel: w268 -> [w270]
              tunnel: [w270] -> w269
              frame #0 {
                w273 = T9 5 items=["Behavior 0", "Behavior 1", "Behavior 2", "Behavior 3", "Behavior 4", "Behavior 5", "Behavior 6"] ("Ring")
                n190 = local read "Behavior Wires In"() -> (w275:T2)
                n191 = Index Array(array=w275, index=w273) -> (element=w278:T1)
                n192 = local read "Behavior Wire In"() -> (w277:T1)
                n193 = Unbundle By Name(w278) -> ("Control Granted"=w271:bool)
                n194 = Bundle By Name(cluster=w277, "Control Granted"=w271, "Control Required"=FALSE) -> (w274:T1)
                n195 = Replace Array Subset(array=w275, new element=w274, index=w273) -> (w272:T2)
                n196 = local write "Behavior Wires In"(w272) -> ()
              }
            }
            n197 = call "Behavior Wires Free.vi"("Sequence In"=w269, "Semaphore Number"=w267) -> ()  [unwired: 8 in, 1 out]
          }
          frame True {
            w279 = T6 0 items=["Motors", "Exit", "Sonar"] ("Semaphores")
            w280 = T6 0 items=["Motors", "Exit", "Sonar"] ("Semaphores")
            # "Trigger condition has been  met so set 'Control Required' Flag and execute behavior if 'Control Granted' flag for Behavior 5 is set."
            n198 = call "Behavior Wires Busy.vi"("Semaphore Number"=w280) -> ("Sequence Out"=w283:T7)  [unwired: 9 in]
            n199 = flat-sequence {
              tunnel: w283 -> [w285]
              tunnel: [w285] -> w282
              tunnel: [w284] -> w281
              frame #0 {
                w291 = T9 5 items=["Behavior 0", "Behavior 1", "Behavior 2", "Behavior 3", "Behavior 4", "Behavior 5", "Behavior 6"] ("Ring")
                # "Step 2: Since trigger Condition has been met, set the 'Control Required' flag for this behavior"
                n200 = local read "Behavior Wires In"() -> (w289:T2)
                n201 = Index Array(array=w289, index=w291) -> (element=w287:T1)
                n202 = local read "Behavior Wire In"() -> (w288:T1)
                n203 = Unbundle By Name(w287) -> ("Control Granted"=w284:bool)
                n204 = Bundle By Name(cluster=w288, "Control Required"=TRUE ("Control Granted"), "Control Granted"=w284) -> (w290:T1)
                n205 = Replace Array Subset(array=w289, new element=w290, index=w291) -> (w292:T2)
                n206 = local write "Behavior Wires In"(w292) -> ()
              }
            }
            n207 = call "Behavior Wires Free.vi"("Sequence In"=w282, "Semaphore Number"=w279) -> ()  [unwired: 8 in, 1 out]
            n208 = case shown="True" w281 {
              frame False {
                # "Control has NOT been granted to this Behavior, so do nothing."
              }
              frame True {
                w294 = i16 7 items=["1", "2", "3", "4", "5", "6", "7", "8", "9", "10", "11", "12"] ("Line")
                w297 = T10 3 items=["Port A"=0, "Port B"=1, "Port C"=2, "Ports A & B"=4, "Ports A & C"=5, "Ports B & C"=6, "All Ports"=3] ("Port (All Ports)")
                # "Your code for Behavior 5 replaces the code here"
                n209 = call-poly <vilib>:"PolyDisplay.vi"("number"=5, "Line"=w294) -> ("NXT/EV3"=w296:T7)  [unwired: 2 in]
                n210 = while {
                  tunnel: w296 -> [w307]
                  tunnel: [w307] -> w293
                  i -> [w305]
                  stop <- w308 stop-if-true
                  w312 = T8 2 items=["Port 1", "Port 2", "Port 3", "Port 4"] ("Port (Port 3)")
                  w316 = T8 3 items=["Port 1", "Port 2", "Port 3", "Port 4"] ("Port (Port 4)")
                  n211 = Multiply(x=6.283185307179586, y=w305) -> (x*y=w304:dbl)
                  n212 = call <vilib>:"Wait_Num(msec).vi"("Time (100 msec)"=u32 200 ("Time (msec)")) -> ()  [unwired: 3 in, 1 out]
                  n213 = call-poly <vilib>:"PolySensor.vi"("Port (Port 3)"=w312) -> ("Detected Color"=w311:T5)  [unwired: 2 in, 1 out]
                  n214 = Divide(x=w304, y=30 ("x")) -> (x/y=w302:dbl)
                  n215 = call-poly <vilib>:"PolySensor.vi"("Port (Port 4)"=w316) -> ("Distance (cm)"=w315:i16)  [unwired: 2 in, 1 out]
                  n216 = call <vilib>:"sine.vi"("x"=w302) -> ("sin(x)"=w319:sgl)
                  n217 = xnode "Motors"() -> ("Motor"=w298:cluster{"Port":T4, "Port":T4})
                  n218 = Not Equal?(x=w311, y=ColorSensorColors."Red") -> (x != y?=w309:bool)
                  n219 = Multiply(x=w319, y=sgl 25.0) -> (x*y=w301:sgl)
                  n220 = Greater?(x=w315, y=i16 254) -> (0:w313:bool)
                  n221 = And(x=w313, y=w309) -> (x .and. y?=w308:bool)
                  n222 = To Word Integer(number=w301) -> (16bit integer=w300:i16)
                  n223 = xnode "LEGO Steering On"("Steering 1"=w300, "Power 1"=50 ("Power (75)"), "Motors"=w298) -> ()  [unwired: 1 in, 1 out]
                }
                n224 = call-poly <vilib>:"PolyMotor.vi"("NXT/EV3"=w293, "Port (All Ports)"=w297) -> ()  [unwired: 3 out]
              }
            }
          }
        }
        n225 = call-poly <vilib>:"NXTFlag_Get_Poly.vi"("NXT/EV3 Flag Number"=w264) -> ("status"=w265:bool)  [unwired: 2 in, 1 out]
      }
      n226 = while {
        stop <- w334 stop-if-true
        w331 = T8 2 items=["Port 1", "Port 2", "Port 3", "Port 4"] ("Port (Port 3)")
        w333 = T6 1 items=["Motors", "Exit", "Sonar"] ("Semaphores")
        # "Behavior 3"
        n227 = call-poly <vilib>:"PolySensor.vi"("Port (Port 3)"=w331) -> ("Detected Color"=w330:T5)  [unwired: 2 in, 1 out]
        n228 = Equal?(x=w330, y=ColorSensors_Enum."Yellow" ("ColorSensor Colours")) -> (x = y?=w329:bool)
        n229 = case shown="True" w329 {
          frame False {
            w335 = T6 0 items=["Motors", "Exit", "Sonar"] ("Semaphores")
            w336 = T6 0 items=["Motors", "Exit", "Sonar"] ("Semaphores")
            # "Trigger Condition has NOT been met so reset the 'Control Required' flag for Behavior 0."
            n230 = call "Behavior Wires Busy.vi"("Semaphore Number"=w335) -> ("Sequence Out"=w337:T7)  [unwired: 9 in]
            n231 = flat-sequence {
              tunnel: w337 -> [w339]
              tunnel: [w339] -> w338
              frame #0 {
                w342 = T9 3 items=["Behavior 0", "Behavior 1", "Behavior 2", "Behavior 3", "Behavior 4", "Behavior 5", "Behavior 6"] ("Ring")
                # "Reset the 'Control Required' Flag"
                n232 = local read "Behavior Wires In"() -> (w344:T2)
                n233 = Index Array(array=w344, index=w342) -> (element=w347:T1)
                n234 = Unbundle By Name(w347) -> ("Control Granted"=w340:bool)
                n235 = local read "Behavior Wire In"() -> (w346:T1)
                n236 = Bundle By Name(cluster=w346, "Control Granted"=w340, "Control Required"=FALSE) -> (w343:T1)
                n237 = Replace Array Subset(array=w344, new element=w343, index=w342) -> (w341:T2)
                n238 = local write "Behavior Wires In"(w341) -> ()
              }
            }
            n239 = call "Behavior Wires Free.vi"("Sequence In"=w338, "Semaphore Number"=w336) -> ()  [unwired: 8 in, 1 out]
          }
          frame True {
            w348 = T6 0 items=["Motors", "Exit", "Sonar"] ("Semaphores")
            w349 = T6 0 items=["Motors", "Exit", "Sonar"] ("Semaphores")
            # "Trigger condition has been  met so set 'Control Required' Flag and execute behavior if 'Control Granted' flag for Behavior 3 is set."
            n240 = call "Behavior Wires Busy.vi"("Semaphore Number"=w349) -> ("Sequence Out"=w352:T7)  [unwired: 9 in]
            n241 = flat-sequence {
              tunnel: w352 -> [w354]
              tunnel: [w354] -> w351
              tunnel: [w353] -> w350
              frame #0 {
                w360 = T9 3 items=["Behavior 0", "Behavior 1", "Behavior 2", "Behavior 3", "Behavior 4", "Behavior 5", "Behavior 6"] ("Ring")
                # "Step 2: Since trigger Condition has been met, set the 'Control Required' flag for this behavior"
                n242 = local read "Behavior Wires In"() -> (w358:T2)
                n243 = Index Array(array=w358, index=w360) -> (element=w356:T1)
                n244 = local read "Behavior Wire In"() -> (w357:T1)
                n245 = Unbundle By Name(w356) -> ("Control Granted"=w353:bool)
                n246 = Bundle By Name(cluster=w357, "Control Required"=TRUE ("Control Granted"), "Control Granted"=w353) -> (w359:T1)
                n247 = Replace Array Subset(array=w358, new element=w359, index=w360) -> (w361:T2)
                n248 = local write "Behavior Wires In"(w361) -> ()
              }
            }
            n249 = call "Behavior Wires Free.vi"("Sequence In"=w351, "Semaphore Number"=w348) -> ()  [unwired: 8 in, 1 out]
            n250 = case shown="True" w350 {
              frame False {
                # "Control has NOT been granted to this Behavior, so do nothing."
              }
              frame True {
                w370 = i16 7 items=["1", "2", "3", "4", "5", "6", "7", "8", "9", "10", "11", "12"] ("Line")
                # "Your code for Behavior 3 replaces the code here"
                n251 = call <vilib>:"RandomNumber.vi"("Max Value"=u16 5) -> ("Random Number"=w368:u16)  [unwired: 2 in, 1 out]
                n252 = xnode "Motors"() -> ("Motor"=w378:cluster{"Port":T4, "Port":T4})
                n253 = call <vilib>:"RandomNumber.vi"("Max Value"=u16 90) -> ("Random Number"=w365:u16)  [unwired: 2 in, 1 out]
                n254 = Add(x=w368, y=u16 5) -> (x+y=w362:u16)
                n255 = local write "Wander Time"(w362) -> ()
                n256 = call-poly <vilib>:"PolyDisplay.vi"("number"=3, "Line"=w370) -> ("NXT/EV3"=w372:T7)  [unwired: 2 in]
                n257 = Add(x=w365, y=u16 90) -> (x+y=w363:u16)
                n258 = local write "Wander Angle"(w363) -> ()
                n259 = xnode "Move Motors"("Power/Speed 2"=i8 25, "Power/Speed 1"=i8 50, "Motors"=w378, "NXT/EV3"=w372) -> ("NXT/EV3"=w373:T7)
                n260 = while {
                  shift-right: [w385] -> w374
                  shift-left: w373 -> [w380]
                  stop <- w381 stop-if-true
                  w382 = T8 0 items=["Port 1", "Port 2", "Port 3", "Port 4"] ("Port (Port 1)")
                  n261 = call-poly <vilib>:"PolyWait.vi"("Time (100 msec)"=u32 100) -> ()  [unwired: 3 in, 1 out]
                  n262 = call-poly <vilib>:"PolySensor.vi"("NXT/EV3"=w380, "Port (Port 3)"=w382) -> ("Detected Color"=w383:T5, "NXT/EV3"=w385:T7)  [unwired: 1 in]
                  n263 = Not Equal?(x=w383, y=ColorSensorColors."Yellow" ("Color (Red)")) -> (x != y?=w381:bool)
                }
                n264 = xnode "Motors"() -> ("Motor"=w375:cluster{"Port":T4, "Port":T4})
                n265 = xnode "Stop Motors"("Motors"=w375, "NXT/EV3"=w374) -> ()  [unwired: 1 out]
              }
            }
          }
        }
        n266 = call-poly <vilib>:"NXTFlag_Get_Poly.vi"("NXT/EV3 Flag Number"=w333) -> ("status"=w334:bool)  [unwired: 2 in, 1 out]
      }
      n267 = while {
        stop <- w404 stop-if-true
        w402 = T8 0 items=["Port 1", "Port 2", "Port 3", "Port 4"] ("Port (Port 1)")
        w403 = T6 1 items=["Motors", "Exit", "Sonar"] ("Semaphores")
        # "Behavior 2"
        n268 = call-poly <vilib>:"PolySensor.vi"("Port (Port 1)"=w402) -> ("Yes / No"=w401:bool)  [unwired: 2 in, 1 out]
        n269 = case shown="True" w401 {
          frame False {
            w405 = T6 0 items=["Motors", "Exit", "Sonar"] ("Semaphores")
            w406 = T6 0 items=["Motors", "Exit", "Sonar"] ("Semaphores")
            # "Trigger Condition has NOT been met so reset the 'Control Required' flag for Behavior 0."
            n270 = call "Behavior Wires Busy.vi"("Semaphore Number"=w405) -> ("Sequence Out"=w407:T7)  [unwired: 9 in]
            n271 = flat-sequence {
              tunnel: w407 -> [w409]
              tunnel: [w409] -> w408
              frame #0 {
                w412 = T9 2 items=["Behavior 0", "Behavior 1", "Behavior 2", "Behavior 3", "Behavior 4", "Behavior 5", "Behavior 6"] ("Ring")
                # "Reset the 'Control Required' Flag"
                n272 = local read "Behavior Wires In"() -> (w414:T2)
                n273 = Index Array(array=w414, index=w412) -> (element=w417:T1)
                n274 = Unbundle By Name(w417) -> ("Control Granted"=w410:bool)
                n275 = local read "Behavior Wire In"() -> (w416:T1)
                n276 = Bundle By Name(cluster=w416, "Control Granted"=w410, "Control Required"=FALSE) -> (w413:T1)
                n277 = Replace Array Subset(array=w414, new element=w413, index=w412) -> (w411:T2)
                n278 = local write "Behavior Wires In"(w411) -> ()
              }
            }
            n279 = call "Behavior Wires Free.vi"("Sequence In"=w408, "Semaphore Number"=w406) -> ()  [unwired: 8 in, 1 out]
          }
          frame True {
            w418 = T6 0 items=["Motors", "Exit", "Sonar"] ("Semaphores")
            w419 = T6 0 items=["Motors", "Exit", "Sonar"] ("Semaphores")
            # "Trigger condition has been  met so set 'Control Required' Flag and execute behavior if 'Control Granted' flag for Behavior 2 is set."
            n280 = call "Behavior Wires Busy.vi"("Semaphore Number"=w419) -> ("Sequence Out"=w422:T7)  [unwired: 9 in]
            n281 = flat-sequence {
              tunnel: w422 -> [w424]
              tunnel: [w424] -> w421
              tunnel: [w423] -> w420
              frame #0 {
                w430 = T9 2 items=["Behavior 0", "Behavior 1", "Behavior 2", "Behavior 3", "Behavior 4", "Behavior 5", "Behavior 6"] ("Ring")
                # "Trigger Condition Met"
                # "Step 2: Since trigger Condition has been met, set the 'Control Required' flag for this behavior"
                n282 = local read "Behavior Wires In"() -> (w428:T2)
                n283 = Index Array(array=w428, index=w430) -> (element=w426:T1)
                n284 = Unbundle By Name(w426) -> ("Control Granted"=w423:bool)
                n285 = local read "Behavior Wire In"() -> (w427:T1)
                n286 = Bundle By Name(cluster=w427, "Control Required"=TRUE ("Control Granted"), "Control Granted"=w423) -> (w429:T1)
                n287 = Replace Array Subset(array=w428, new element=w429, index=w430) -> (w431:T2)
                n288 = local write "Behavior Wires In"(w431) -> ()
              }
            }
            n289 = call "Behavior Wires Free.vi"("Sequence In"=w421, "Semaphore Number"=w418) -> ()  [unwired: 8 in, 1 out]
            n290 = case shown="True" w420 {
              frame False {
                # "Control has NOT been granted to this Behavior, so do nothing."
              }
              frame True {
                w440 = 409 ("x")
                w445 = u16 0 items=["right", "left"] ("Ring")
                w450 = i8 -75 ("Power/Speed 1")
                w453 = i16 7 items=["1", "2", "3", "4", "5", "6", "7", "8", "9", "10", "11", "12"] ("Line")
                # "Your code for Behavior 2 replaces the code here"
                n291 = local read "Wander Direction"() -> (w433:u16)
                n292 = xnode "Motors"() -> ("Motor"=w452:cluster{"Port":T4, "Port":T4})
                n293 = local read "Wander Speed"() -> (w432:i32)
                n294 = Equal?(x=w433, y=w445) -> (x = y?=w444:bool)
                n295 = call <vilib>:"RandomNumber.vi"("Max Value"=u16 90) -> ("Random Number"=w438:u16)  [unwired: 2 in, 1 out]
                n296 = call <vilib>:"RandomNumber.vi"("Max Value"=u16 90) -> ("Random Number"=w437:u16)  [unwired: 2 in, 1 out]
                n297 = call-poly <vilib>:"PolyDisplay.vi"("number"=2, "Line"=w453) -> ("NXT/EV3"=w451:T7)  [unwired: 2 in]
                n298 = Add(x=w438, y=w437) -> (x+y=w436:u16)
                n299 = Select(t=i8 1, s=w444, f=i8 -1) -> (s? t:f=w446:i8)
                n300 = xnode "Move a Fixed Distance"("Speed 2"=w450, "Speed 1"=w450, "Distance 2"=w440, "Distance 1"=w440, "Motors"=w452, "NXT/EV3"=w451) -> ("NXT/EV3"=w443:T7)
                n301 = Multiply(x=w446, y=w432) -> (x*y=w442:i32)
                n302 = Add(x=w436, y=i8 90) -> (x+y=w441:u16)
                n303 = call "Rotate.vi"("Rotation"=w441, "Direction/Speed"=w442, "Input"=w443) -> ("Output"=w434:T7)  [unwired: 8 in]
                n304 = flat-sequence {
                  tunnel: w433 -> [w455]
                  tunnel: w434 -> [_]
                  frame #0 {
                    n305 = case shown="0, Default" w455 {
                      tunnel: [w457 w458] -> w456
                      frame 0, Default {
                        w457 = u16 1 items=["right", "left"] ("Ring")
                      }
                      frame 1 {
                        w458 = u16 0 items=["right", "left"] ("Ring")
                      }
                    }
                    n306 = local write "Wander Direction"(w456) -> ()
                  }
                }
              }
            }
          }
        }
        n307 = call-poly <vilib>:"NXTFlag_Get_Poly.vi"("NXT/EV3 Flag Number"=w403) -> ("status"=w404:bool)  [unwired: 2 in, 1 out]
      }
      n308 = while {
        stop <- w604 stop-if-true
        w603 = T6 1 items=["Motors", "Exit", "Sonar"] ("Semaphores")
        # "Behavior 0"
        n309 = case shown="True" TRUE {
          frame False {
            w605 = T6 0 items=["Motors", "Exit", "Sonar"] ("Semaphores")
            w606 = T6 0 items=["Motors", "Exit", "Sonar"] ("Semaphores")
            # "Trigger Condition has NOT been met so reset the 'Control Required' flag for Behavior 0."
            n310 = call "Behavior Wires Busy.vi"("Semaphore Number"=w605) -> ("Sequence Out"=w607:T7)  [unwired: 9 in]
            n311 = flat-sequence {
              tunnel: w607 -> [w609]
              tunnel: [w609] -> w608
              frame #0 {
                w612 = T9 0 items=["Behavior 0", "Behavior 1", "Behavior 2", "Behavior 3", "Behavior 4", "Behavior 5", "Behavior 6"] ("Ring")
                # "Reset the 'Control Required' Flag"
                n312 = local read "Behavior Wires In"() -> (w614:T2)
                n313 = Index Array(array=w614, index=w612) -> (element=w617:T1)
                n314 = Unbundle By Name(w617) -> ("Control Granted"=w610:bool)
                n315 = local read "Behavior Wire In"() -> (w616:T1)
                n316 = Bundle By Name(cluster=w616, "Control Granted"=w610, "Control Required"=FALSE) -> (w613:T1)
                n317 = Replace Array Subset(array=w614, new element=w613, index=w612) -> (w611:T2)
                n318 = local write "Behavior Wires In"(w611) -> ()
              }
            }
            n319 = call "Behavior Wires Free.vi"("Sequence In"=w608, "Semaphore Number"=w606) -> ()  [unwired: 8 in, 1 out]
          }
          frame True {
            w618 = T6 0 items=["Motors", "Exit", "Sonar"] ("Semaphores")
            w619 = T6 0 items=["Motors", "Exit", "Sonar"] ("Semaphores")
            # "Trigger condition has been  met so set 'Control Required' Flag and execute behavior if 'Control Granted' flag for Behavior 0 is set."
            n320 = call "Behavior Wires Busy.vi"("Semaphore Number"=w619) -> ("Sequence Out"=w622:T7)  [unwired: 9 in]
            n321 = flat-sequence {
              tunnel: w622 -> [w624]
              tunnel: [w624] -> w621
              tunnel: [w623] -> w620
              frame #0 {
                w630 = T9 0 items=["Behavior 0", "Behavior 1", "Behavior 2", "Behavior 3", "Behavior 4", "Behavior 5", "Behavior 6"] ("Ring")
                # "Trigger Condition Met"
                # "Step 2: Since trigger Condition has been met, set the 'Control Required' flag for this behavior"
                n322 = local read "Behavior Wires In"() -> (w628:T2)
                n323 = Index Array(array=w628, index=w630) -> (element=w626:T1)
                n324 = local read "Behavior Wire In"() -> (w627:T1)
                n325 = Unbundle By Name(w626) -> ("Control Granted"=w623:bool)
                n326 = Bundle By Name(cluster=w627, "Control Required"=TRUE ("Control Granted"), "Control Granted"=w623) -> (w629:T1)
                n327 = Replace Array Subset(array=w628, new element=w629, index=w630) -> (w631:T2)
                n328 = local write "Behavior Wires In"(w631) -> ()
              }
            }
            n329 = call "Behavior Wires Free.vi"("Sequence In"=w621, "Semaphore Number"=w618) -> ()  [unwired: 8 in, 1 out]
            n330 = case shown="True" w620 {
              frame False {
                # "Control has NOT been granted to this Behavior, so do nothing."
              }
              frame True {
                w636 = u16 0 items=["left", "right"] ("Ring")
                w638 = T9 0 items=["Behavior 0", "Behavior 1", "Behavior 2", "Behavior 3", "Behavior 4", "Behavior 5", "Behavior 6"] ("Ring")
                w641 = i16 7 items=["1", "2", "3", "4", "5", "6", "7", "8", "9", "10", "11", "12"] ("Line")
                # "Your code for Behavior 0 replaces the code here"
                n331 = local read "Wander Direction"() -> (w637:u16)
                n332 = xnode "Motors"() -> ("Motor"=w650:cluster{"Port":T4, "Port":T4})
                n333 = call-poly <vilib>:"NXTFlag_Assign_Poly.vi"("NXT/EV3 Flag Number"=i8 7) -> ()  [unwired: 3 in, 1 out]
                n334 = local read "Wander Speed"() -> (w635:i32)
                n335 = call-poly <vilib>:"PolyDisplay.vi"("number"=w638, "Line"=w641) -> ("NXT/EV3"=w642:T7)  [unwired: 2 in]
                n336 = local read "Wander Time"() -> (w634:i32)
                n337 = Equal?(x=w637, y=w636) -> (x = y?=w643:bool)
                n338 = xnode "Move Motors"("Power/Speed 2"=w635, "Power/Speed 1"=w635, "Motors"=w650, "NXT/EV3"=w642) -> ("NXT/EV3"=w649:T7)
                n339 = xnode "Motors"() -> ("Motor"=w647:cluster{"Port":T4, "Port":T4})
                n340 = call-poly <vilib>:"PolyWait.vi"("Time (1 sec)"=w634, "NXT/EV3"=w649) -> ("NXT/EV3"=w648:T7)  [unwired: 2 in]
                n341 = local read "Wander Angle"() -> (w633:i32)
                n342 = Select(t=i8 1, s=w643, f=i8 -1) -> (s? t:f=w644:i8)
                n343 = xnode "Stop Motors"("Motors"=w647, "NXT/EV3"=w648) -> ("NXT/EV3"=w640:T7)
                n344 = Multiply(x=w635, y=w644) -> (x*y=w639:i32)
                n345 = call "Rotate.vi"("Rotation"=w633, "Direction/Speed"=w639, "Input"=w640) -> ()  [unwired: 8 in, 1 out]
              }
            }
          }
        }
        n346 = call-poly <vilib>:"NXTFlag_Get_Poly.vi"("NXT/EV3 Flag Number"=w603) -> ("status"=w604:bool)  [unwired: 2 in, 1 out]
      }
      n347 = while {
        shift-right: [w591] -> w18
        shift-left: w17 -> [w590]
        stop <- w593 stop-if-true
        w588 = T11 3 items=["Enter button"=3, "Left button"=2, "Right button"=1, "Up Button"=4, "Down Button"=5] ("Button (Enter button)")
        w589 = T6 1 items=["Motors", "Exit", "Sonar"] ("Semaphores")
        # "This loop permits the program to be terminated by pressing the Orange Button"
        n348 = call-poly <vilib>:"PolyWait.vi"("Time (100 msec)"=u32 100) -> ()  [unwired: 3 in, 1 out]
        n349 = call-poly <vilib>:"PolySensor.vi"("Button (Enter button)"=w588, "NXT/EV3"=w590) -> ("Yes/No"=w595:bool, "NXT/EV3"=w596:T7)  [unwired: 1 in]
        n350 = case shown="True" w595 {
          tunnel: w596 -> [w597 w601]
          tunnel: [w597 w600] -> w594
          frame False {
            # "Shutdown not initiated, so do nothing."
          }
          frame True {
            w598 = T6 1 items=["Motors", "Exit", "Sonar"] ("Semaphores")
            # "Set Exit flag to signal other loops to shutdown."
            n351 = call-poly <vilib>:"NXTFlag_Assign_Poly.vi"("Flag State"=TRUE, "NXT/EV3"=w601, "NXT/EV3 Flag Number"=w598) -> ("NXT/EV3"=w600:T7)  [unwired: 1 in]
          }
        }
        n352 = call-poly <vilib>:"NXTFlag_Get_Poly.vi"("Clear if Found"=FALSE, "NXT/EV3"=w594, "NXT/EV3 Flag Number"=w589) -> ("status"=w593:bool, "NXT/EV3"=w591:T7)
      }
      n353 = while {
        stop <- w26 stop-if-true
        w25 = T6 1 items=["Motors", "Exit", "Sonar"] ("Semaphores")
        n354 = call-poly <vilib>:"NXTFlag_Get_Poly.vi"("NXT/EV3 Flag Number"=7) -> ("status"=w24:bool, "NXT/EV3"=w20:T7)  [unwired: 2 in]
        n355 = call-poly <vilib>:"PolyWait.vi"("Time (100 msec)"=u32 100) -> ()  [unwired: 3 in, 1 out]
        n356 = case shown="True" w24 {
          tunnel: [w27 w28] -> w21
          tunnel: w20 -> [w27 w30]
          frame False {
          }
          frame True {
            n357 = call-poly <vilib>:"PolyWait.vi"("Time (100 msec)"=u32 5000, "NXT/EV3"=w30) -> ("NXT/EV3"=w29:T7)  [unwired: 2 in]
            n358 = call-poly <vilib>:"PolySound.vi"("Duration (500 ms)"=u16 250, "NXT/EV3"=w29) -> ("NXT/EV3"=w28:T7)  [unwired: 2 in]
          }
        }
        n359 = call-poly <vilib>:"NXTFlag_Get_Poly.vi"("NXT/EV3 Flag Number"=w25) -> ("status"=w26:bool)  [unwired: 2 in, 1 out]
        n360 = call-poly <vilib>:"NXTFlag_Clear_Poly.vi"("NXT/EV3"=w21, "NXT/EV3 Flag Number"=7) -> ()  [unwired: 2 in, 1 out]
      }
    }
    frame #2 {
      w681 = i16 7 items=["1", "2", "3", "4", "5", "6", "7", "8", "9", "10", "11", "12"] ("Line")
      # "Step 3: \n\nShutdown operations"
      n361 = call-poly <vilib>:"PolyDisplay.vi"("number"=6, "NXT/EV3"=w666, "Line"=w681) -> ("NXT/EV3"=w679:T7)  [unwired: 1 in]
      n362 = call-poly <vilib>:"PolySound.vi"("Duration (500 ms)"=u16 500, "NXT/EV3"=w679, "Tone (440 Hz)"=u16 440) -> ("NXT/EV3"=w678:T7)  [unwired: 1 in]
      n363 = call-poly <vilib>:"PolySound.vi"("Duration (500 ms)"=u16 500, "NXT/EV3"=w678, "Tone (440 Hz)"=u16 350) -> ("NXT/EV3"=w677:T7)  [unwired: 1 in]
      n364 = call-poly <vilib>:"PolySound.vi"("Duration (500 ms)"=u16 250, "NXT/EV3"=w677, "Tone (440 Hz)"=u16 440) -> ("NXT/EV3"=w676:T7)  [unwired: 1 in]
      n365 = call-poly <vilib>:"PolySound.vi"("Duration (500 ms)"=u16 250, "NXT/EV3"=w676, "Tone (440 Hz)"=u16 554) -> ("NXT/EV3"=w675:T7)  [unwired: 1 in]
      n366 = call "Rotate.vi"("Rotation"=i16 720, "Input"=w675) -> ()  [unwired: 9 in, 1 out]
    }
  }
